vi "dmm_measurement.vi"(4 "Sequence Context":T1) -> (0 "error out":errorcluster, 1 "Test Data":T2 {"Numeric Measurement" format="%.2f"})   [LabVIEW 2012]
uses:
  <vilib>/addons/TestStand/_TSUtility.llb/TestStand - Get Property Value (String).vi
  Demo/LabVIEW/SupportVIs.llb/LabVIEW Test - Test Data.ctl
  <vilib>/addons/TestStand/_TSLegacy.llb/LabVIEW Test - Sequence Context.ctl
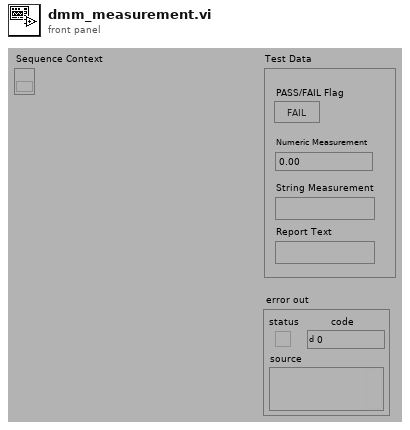
[diagram p1: front panel]
types:
  T1 = typedef "LabVIEW Test - Sequence Context.ctl" = refnum<k7>
  T2 = typedef "LabVIEW Test - Test Data.ctl" = cluster{"PASS/FAIL Flag":bool, "Numeric Measurement":dbl, "String Measurement":string, "Report Text":string}
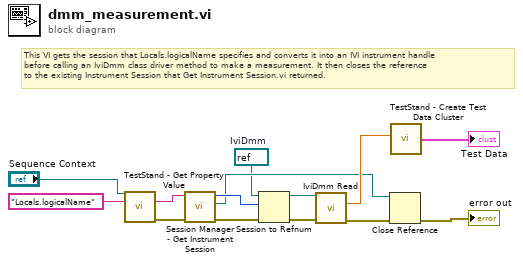
[diagram p0: block diagram]
diagram:
  w1 = refnum<k15> refnum  # IviDmm
  # "This VI gets the session that Locals.logicalName specifies and converts it into an IVI instrument handle\nbefore calling an IviDmm class driver method to make a measurement. It then closes the reference\nto the existing Instrument Session that Get Instrument Session.vi returned."
  n1 = call-poly <vilib>:"TestStand - Get Property Value.vi"("Sequence Context In"="Sequence Context", "Lookup String"="Locals.logicalName") -> ("Value"=w5:string, "error out"=w7:errorcluster)  [unwired: 1 in, 11 out]
  n2 = call <vilib>:"Session Manager - Get Instrument Session.vi"("error in (no error)"=w7, "Session Name"=w5) -> ("error out"=w12:errorcluster, "Instrument Session"=w2:refnum<k7>, "Driver Handle"=w13:u32)  [unwired: 1 in, 6 out]
  n3 = Session to Refnum(4:w12, 6:w13, 7:w1) -> (0:w11:errorcluster, 3:w10:refnum<k15>)
  n4 = call <vilib>:"IviDmm Read.vi"("error in (no error)"=w11, "instrument handle"=w10) -> ("error out"=w4:errorcluster, "reading"=w9:dbl)  [unwired: 1 in, 7 out]
  n5 = Close Reference(reference=w2, error in (no error)=w4) -> (error out=→"error out":errorcluster)
  n6 = call "TestStand - Create Test Data Cluster.vi"("Numeric Measurement"=w9) -> ("Test Data"=→"Test Data":T2)  [unwired: 3 in]
